vi "发送字符串.vi"(11 "字符串":string) -> (3 "连接的字符串 2":string)   [LabVIEW 2012]
panel:
  out "添加的数组":string[](array[string])
  out "无符号8位整型":u8[](array[numeric]) format="%x"
  out "CRCLo":u8 format="%x"
  out "CRCHi":u8 format="%x"
  out "十六进制整型字符串":string[](array[string])
  out "十六进制整型字符串 2":string[](array[string])
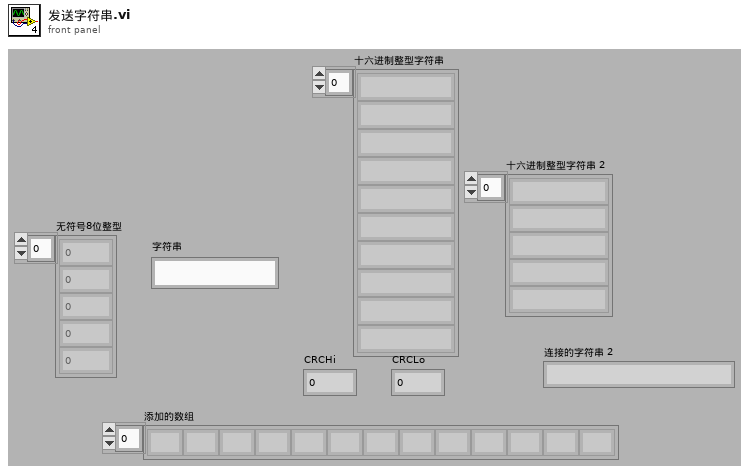
[diagram p1: front panel]
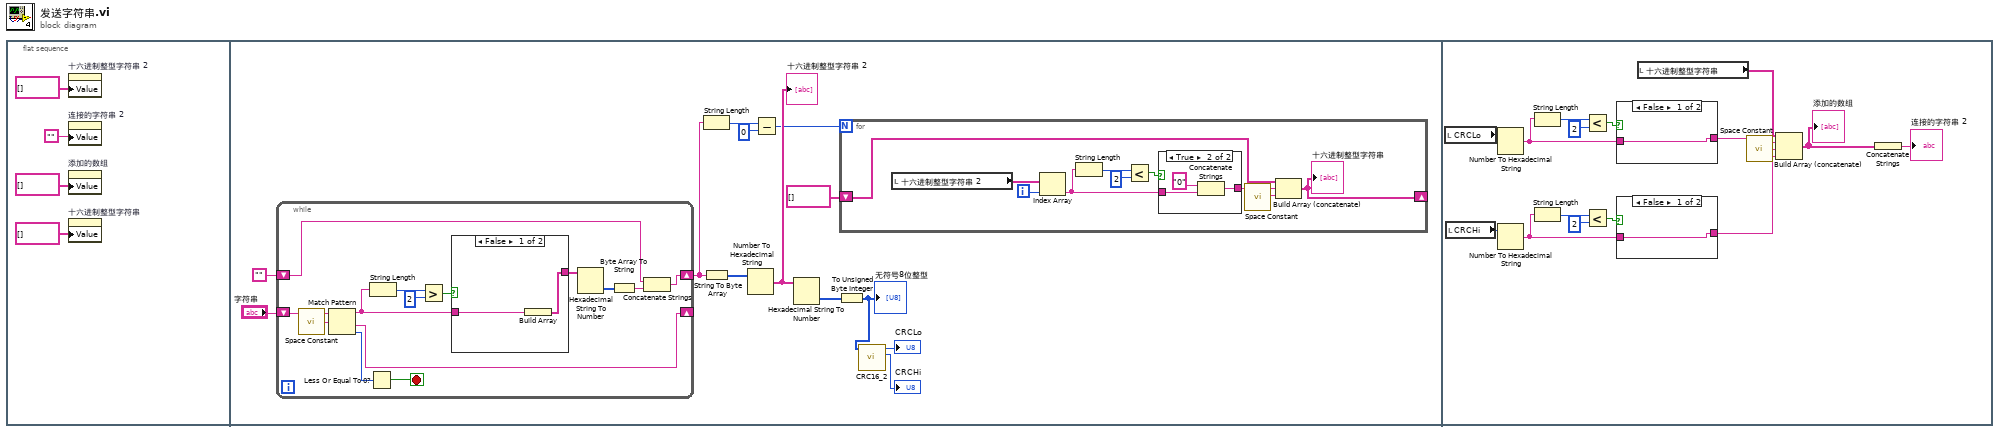
[diagram p0: block diagram]
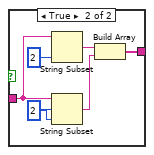
[diagram p3: hidden frame]
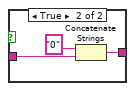
[diagram p4: hidden frame]
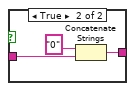
[diagram p5: hidden frame]
diagram:
  n1 = flat-sequence {
    frame #0 {
      n2 = property on="十六进制整型字符串 2" class="Arr (strict)"("Value"=string[] [] ("十六进制整型字符串 2")) -> ()  [unwired: 2 in, 2 out]
      n3 = property on="连接的字符串 2" class="Str"("Value"="") -> ()  [unwired: 2 in, 2 out]
      n4 = property on="添加的数组" class="Arr (strict)"("Value"=string[] [] ("添加的数组")) -> ()  [unwired: 2 in, 2 out]
      n5 = property on="十六进制整型字符串" class="Arr (strict)"("Value"=string[] [] ("十六进制整型字符串")) -> ()  [unwired: 2 in, 2 out]
    }
    frame #1 {
      n6 = while {
        shift-right: [w44] -> _
        shift-left: "字符串" -> [w45]
        shift-right: [w39] -> w14
        shift-left: "" -> [w41]
        stop <- w37 stop-if-true
        n7 = call <vilib>:"Space Constant.vi"() -> ("String"=w43:string)
        n8 = Match Pattern(string=w45, regular expression=w43) -> (before substring=w33:string, after substring=w44:string, offset past match=w38:i32)  [unwired: 2 out]
        n9 = Less Or Equal To 0?(x=w38) -> (x <= 0?=w37:bool)
        n10 = String Length(string=w33) -> (length=w36:i32)
        n11 = Greater?(x=w36, y=2) -> (0:w34:bool)
        n12 = case shown="False" w34 {
          tunnel: w33 -> [w47 w52]
          tunnel: [w46 w48] -> w32
          frame False {
            n13 = Build Array(w47) -> (w46:string[])
          }
          frame True {
            w51 = 2 ("偏移量(0)")
            n14 = String Subset(string=w52, length (rest)=2 ("长度（剩余）")) -> (substring=w50:string)  [unwired: 1 out]
            n15 = String Subset(string=w52, offset (0)=w51, length (rest)=w51) -> (substring=w49:string)
            n16 = Build Array(w50, w49) -> (w48:string[])
          }
        }
        n17 = Hexadecimal String To Number(string=w32) -> (number=w42:u32[])  [unwired: 3 out]
        n18 = Byte Array To String(unsigned byte array=w42) -> (string=w40:string)
        n19 = Concatenate Strings(w41, w40) -> (w39:string)
      }
      n20 = String Length(string=w14) -> (length=w10:i32)
      n21 = String To Byte Array(string=w14) -> (unsigned byte array=w16:u8[])
      n22 = Number To Hexadecimal String(2:w16) -> (0:w13:string[])  [unwired: 1 out]
      "十六进制整型字符串 2" <- w13
      n23 = Subtract(x=w10, y=0) -> (x-y=w8:i32)
      n24 = Hexadecimal String To Number(string=w13) -> (number=w15:u32[])  [unwired: 3 out]
      n25 = To Unsigned Byte Integer(number=w15) -> (unsigned 8bit integer=w7:u8[])
      "无符号8位整型" <- w7
      n26 = for {
        N: w8 -> [_]
        shift-right: [w18] -> _
        shift-left: string[] [] -> [w21]
        i -> [w22]
        n27 = local read "十六进制整型字符串 2"() -> (w24:string[])
        n28 = Index Array(array=w24, index=w22) -> (element=w23:string)
        n29 = String Length(string=w23) -> (length=w27:i32)
        n30 = Less?(x=w27, y=2) -> (x < y?=w25:bool)
        n31 = case shown="True" w25 {
          tunnel: [w28 w30] -> w20
          tunnel: w23 -> [w28 w29]
          frame False {
          }
          frame True {
            n32 = Concatenate Strings("0" ("字符串"), w29) -> (w30:string)
          }
        }
        n33 = call <vilib>:"Space Constant.vi"() -> ("String"=w19:string)
        n34 = Build Array (concatenate)(w21, w20, w19) -> (w18:string[])
        "十六进制整型字符串" <- w18
      }
      n35 = call "CRC16_2.vi"("buf"=w7) -> ("CRCHi"=→"CRCHi":u8, "CRCLo"=→"CRCLo":u8)  [unwired: 9 in]
    }
    frame #2 {
      n36 = local read "CRCLo"() -> (w69:u8)
      n37 = local read "CRCHi"() -> (w62:u8)
      n38 = Number To Hexadecimal String(2:w69) -> (0:w55:string)  [unwired: 1 out]
      n39 = Number To Hexadecimal String(2:w62) -> (0:w60:string)  [unwired: 1 out]
      n40 = String Length(string=w55) -> (length=w58:i32)
      n41 = String Length(string=w60) -> (length=w64:i32)
      n42 = Less?(x=w58, y=2) -> (x < y?=w56:bool)
      n43 = Less?(x=w64, y=2) -> (x < y?=w61:bool)
      n44 = case shown="False" w56 {
        tunnel: w55 -> [w70 w72]
        tunnel: [w70 w71] -> w54
        frame False {
        }
        frame True {
          n45 = Concatenate Strings("0" ("字符串"), w72) -> (w71:string)
        }
      }
      n46 = case shown="False" w61 {
        tunnel: w60 -> [w74 w76]
        tunnel: [w74 w75] -> w59
        frame False {
        }
        frame True {
          n47 = Concatenate Strings("0" ("字符串"), w76) -> (w75:string)
        }
      }
      n48 = local read "十六进制整型字符串"() -> (w68:string[])
      n49 = call <vilib>:"Space Constant.vi"() -> ("String"=w67:string)
      n50 = Build Array (concatenate)(w68, w54, w67, w59) -> (w66:string[])
      "添加的数组" <- w66
      n51 = Concatenate Strings(w66) -> (→"连接的字符串 2":string)
    }
  }
